vi "Create Server Sent Event Resource.vi"(8 "error in (no error)":errorcluster, 9 "SSE Manager":refnum<class "SSE Manager.lvclass">, 10 "Path":string, 11 "Server in":refnum<class "Server.lvclass">) -> (0 "error out":errorcluster, 3 "Server out":refnum<class "Server.lvclass">)   [LabVIEW 2020, in "HTTP Server.lvlib" / "Server.lvclass"]
uses:
  Server.lvclass
  SSE Manager/SSE Manager.lvclass
  Server.lvclass/Server.ctl
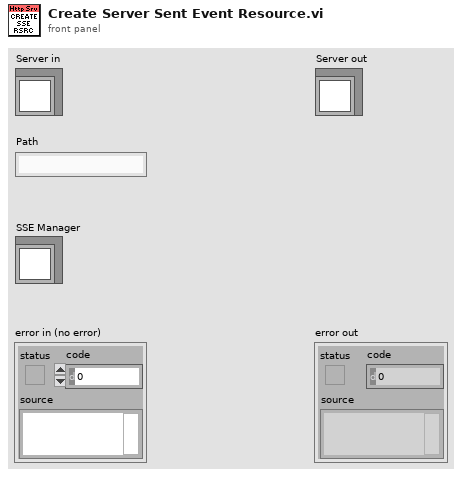
[diagram p1: front panel]
types:
  T1 = typedef "HTTP Server.lvlib/Server Sent Events Data.ctl" = cluster{"Resources":map{string, refnum<class "SSE Manager.lvclass">}}
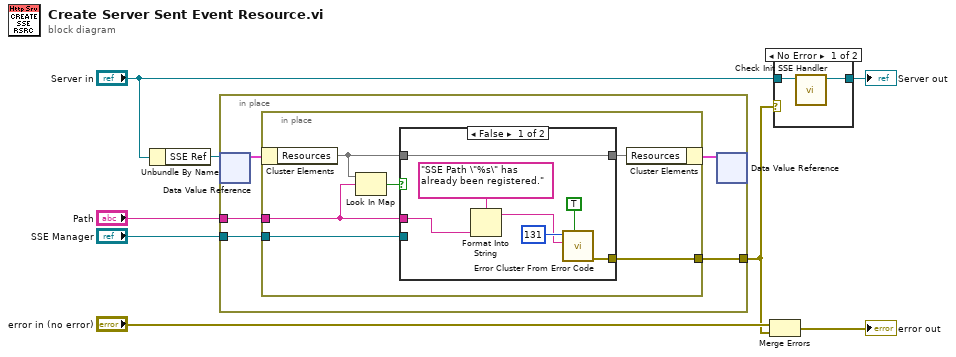
[diagram p0: block diagram]
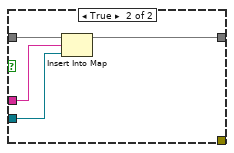
[diagram p2: hidden frame]
diagram:
  n1 = Unbundle By Name("Server in") -> ("SSE Ref"=w7:refnum<data-value>)
  n2 = in-place {
    in-place-border: "Path" -> [w11]
    in-place-border: "SSE Manager" -> [w10]
    in-place-border: [w9] -> w1
    n3 = in-place-dvr #1(w7) -> (w13:T1)  [unwired: 1 out]
    n4 = in-place {
      in-place-border: w11 -> [w16]
      in-place-border: w10 -> [w17]
      in-place-border: [w14] -> w9
      n5 = in-place-cluster #2(w13) -> ("Resources"=w18:map{string, refnum<class "SSE Manager.lvclass">})
      n6 = Look In Map(map=w18, key=w16) -> (key not found?=w19:bool)  [unwired: 1 in, 1 out]
      n7 = case shown="False" w19 {
        tunnel: w18 -> [w26 w30]
        tunnel: w17 -> [_ w29]
        tunnel: w16 -> [w22 w28]
        tunnel: [w26 w27] -> w15
        tunnel: [w20 _] -> w14
        frame False {
          n8 = Format Into String(format string="SSE Path \"%s\" has already been registered.", w22) -> (resulting string=w21:string)  [unwired: 2 in, 1 out]
          n9 = call <vilib>:"Error Cluster From Error Code.vi"("show call chain? (False)"=TRUE, "error message (\"\")"=w21, "error code (0)"=131) -> ("error out"=w20:errorcluster)  [unwired: 6 in]
        }
        frame True {
          n10 = Insert Into Map(map in=w30, key=w28, value=w29) -> (map out=w27:map{string, refnum<class "SSE Manager.lvclass">})  [unwired: 2 out]
        }
      }
      n11 = in-place-cluster #2("Resources"=w15) -> (w12:T1)
    }
    n12 = in-place-dvr #1(w12) -> ()  [unwired: 2 out]
  }
  n13 = Merge Errors("error in (no error)", w1) -> (→"error out":errorcluster)
  n14 = case shown="No Error" w1 {
    tunnel: "Server in" -> [w32 w33]
    tunnel: [w31 w33] -> w3
    frame No Error {
      n15 = call "Check Init SSE Handler.vi"("Server in"=w32) -> ("Server out"=w31:refnum<class "Server.lvclass">)  [unwired: 9 in, 1 out]
    }
    frame Error {
    }
  }
  "Server out" <- w3
